vi "2D ANOVA.vi"(6 "B levels":i32 format="%0.0f", 7 "A levels":i32 format="%0.0f", 8 "observations per cell":i32=1 format="%0.0f", 9 "Index B":i32[](array[numeric]) format="%0.0f", 10 "Index A":i32[](array[numeric]) format="%0.0f", 11 "X":dbl[](array[numeric]) format="%0.4f") -> (0 "sig AB":dbl format="%0.10f", 1 "sig B":dbl format="%0.10f", 2 "sig A":dbl format="%0.10f", 3 "Info":dbl[][](array[numeric]) format="%0.4f", 4 "error":i32)   [LabVIEW 2017, in "NI_AALPro.lvlib"]
doc: "Takes an array of experimental observations made at various levels of two factors and performs a two-way analysis of variance."
uses:
  NI_AALPro.lvlib
  <resource>/lvanlys.dll
panel:
  # "2D ANOVA"
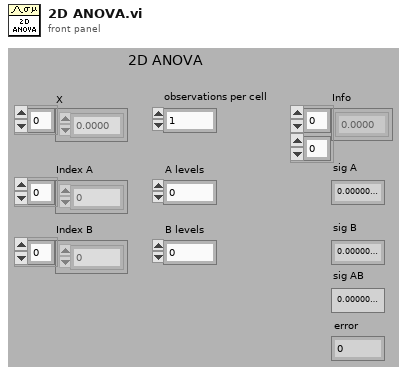
[diagram p1: front panel]
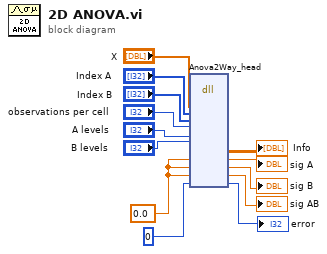
[diagram p0: block diagram]
diagram:
  w10 = 0.0
  n1 = dll-call lib="C:/Program Files (x86)/National Instruments/LabVIEW 2017/resource/lvanlys.*" fn="Anova2Way_head"("X"="X", "Index A"="Index A", "Index B"="Index B", "observations per cell"="observations per cell", "A levels"="A levels", "B levels"="B levels", w10, w10, w10, 0) -> ("Info"=→"Info":dbl[][], →"sig A":dbl, →"sig B":dbl, →"sig AB":dbl, →"error":i32)  [unwired: 11 in, 2 out]
